vi "NI VeriStand - Get Aliases.vi"(8 "Error in":errorcluster, 11 "Runtime Configuration Ref in":refnum<k24>) -> (0 "Error out":errorcluster, 1 "Alias Names":string[](array[string]), 2 "Referenced Channels":string[](array[string]), 3 "Runtime Configuration Ref out":refnum<k24>, 4 "Success":bool, 5 "Runtime Alias Folder Name":string)   [LabVIEW 2025, in "NI_VS RuntimeConfigurationFile ScriptingAPI.lvlib"]
uses:
  NI_VS RuntimeConfigurationFile ScriptingAPI.lvlib
  NationalInstruments.VeriStand.SystemDefinitionAPI
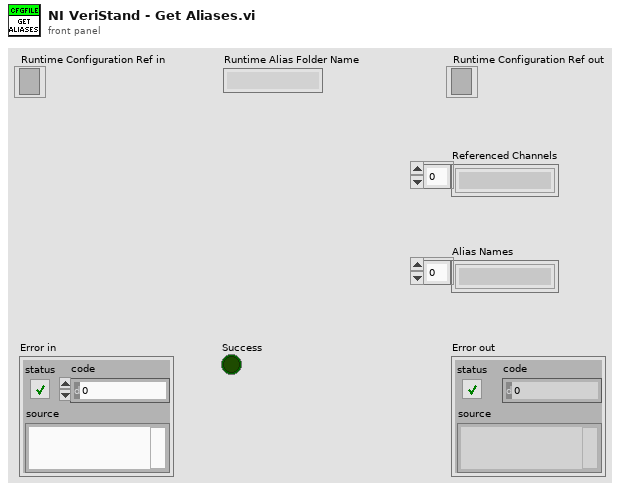
[diagram p1: front panel]
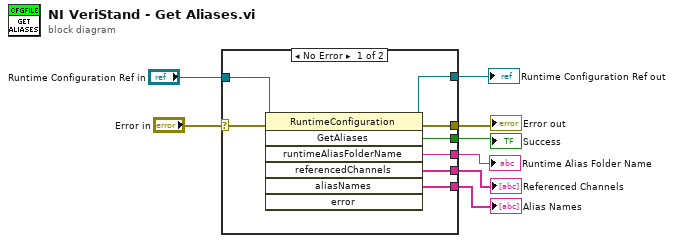
[diagram p0: block diagram]
diagram:
  n1 = case shown="No Error" "Error in" {
    selector: "Error in" -> [w15 w17]
    tunnel: "Runtime Configuration Ref in" -> [w14 _]
    tunnel: [w13 _] -> w5
    tunnel: [w16 w17] -> w8
    tunnel: [w12 _] -> w4
    tunnel: [w11 _] -> w3
    tunnel: [w10 _] -> w2
    tunnel: [w9 _] -> w1
    frame No Error {
      n2 = invoke class="RuntimeConfiguration" method="GetAliases"(reference=w14, error in=w15) -> (reference out=w13:refnum<k24>, error out=w16:errorcluster, "GetAliases"=w12:bool, "runtimeAliasFolderName"=w9:string, "referencedChannels"=w11:string[], "aliasNames"=w10:string[])  [unwired: 5 in, 1 out]
    }
    frame Error {
    }
  }
  "Runtime Configuration Ref out" <- w5
  "Error out" <- w8
  "Success" <- w4
  "Referenced Channels" <- w3
  "Alias Names" <- w2
  "Runtime Alias Folder Name" <- w1
